vi "GetControllerTemp.vi"(8 "error in (no error)":errorcluster, 11 "SM1000-control in":T1) -> (0 "error out":errorcluster, 2 "Controller temperature":dbl, 3 "SM1000-control out":T1)   [LabVIEW 2013, in "SLMControl.lvlib" / "SM1000.lvclass"]
doc: "Returns the current temperature of the EC1000 board in degrees Celsius.\n\nCommand: \"GetControllerTemp\" or 29\nReturns: floats"
uses:
  SM1000.lvclass
  Object-reference.ctl
  SM1000.lvclass/SM1000.ctl
  Custom-errors.ctl
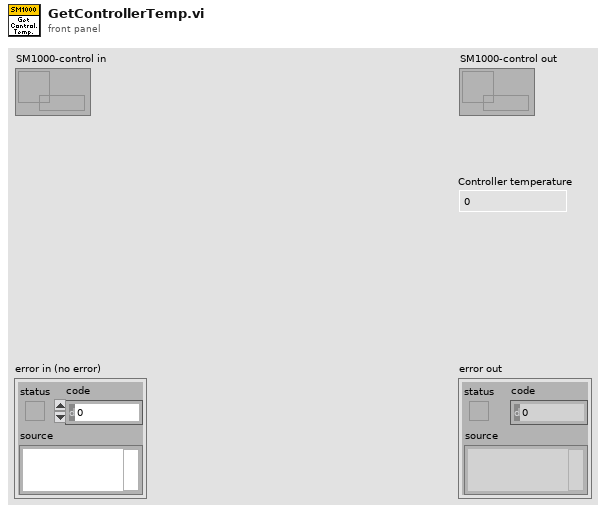
[diagram p1: front panel]
types:
  T1 = typedef "SLMControl.lvlib/SM1000.lvclass/Object-reference.ctl" = refnum<data-value>
  T2 = typedef "SLMControl.lvlib/SM1000.lvclass/Custom-errors.ctl" = enum16{"No error", "Not implemented", "Command not recognized", "Invalid input", "No connection", "Timeout", "Resource not loaded"}
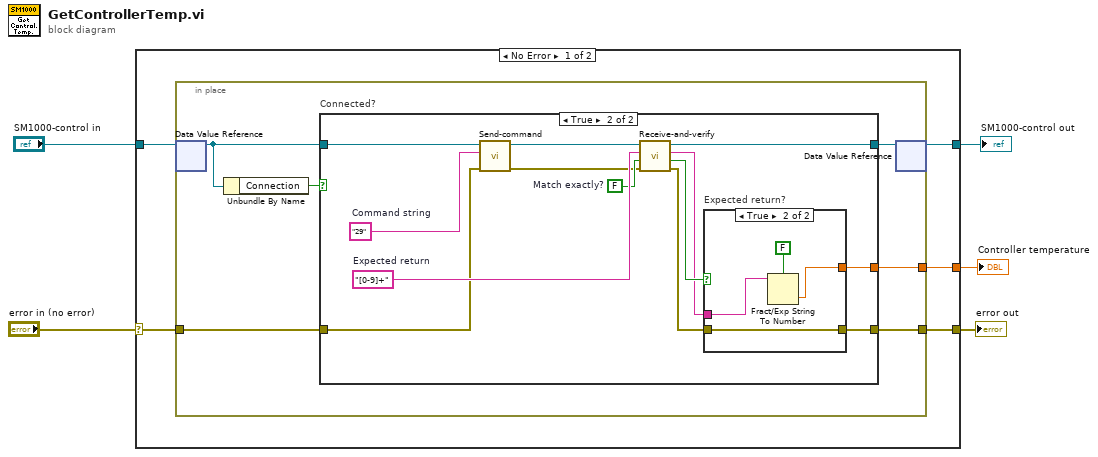
[diagram p0: block diagram]
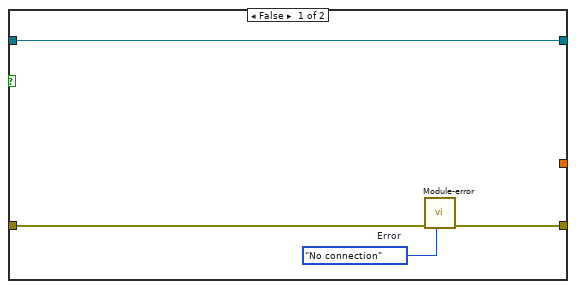
[diagram p2: hidden frame]
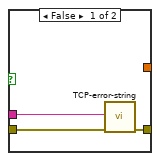
[diagram p3: hidden frame]
diagram:
  n1 = case shown="No Error" "error in (no error)" {
    selector: "error in (no error)" -> [w8 w42]
    tunnel: [w7 w42] -> w4
    tunnel: [w9 w41] -> w2
    tunnel: "SM1000-control in" -> [w10 w41]
    tunnel: [w6 _] -> w1
    frame No Error {
      n2 = in-place {
        in-place-border: w8 -> [w16]
        in-place-border: [w13] -> w7
        in-place-border: [w11] -> w6
        n3 = in-place-dvr #1(w10) -> (w14:refnum<class "SM1000.lvclass">)  [unwired: 1 out]
        n4 = Unbundle By Name(w14) -> ("Connection"=w15:bool)
        n5 = case "Connected?" shown="True" w15 {
          tunnel: w16 -> [w20 w25]
          tunnel: w14 -> [w18 w33]
          tunnel: [w19 w23] -> w13
          tunnel: [w18 w22] -> w12
          tunnel: [_ w21] -> w11
          frame False {
            w17 = Custom-errors."No connection"  # Error
            n6 = call "Module-error.vi"("Error"=w17, "error in (no error)"=w20) -> ("error out"=w19:errorcluster)  [unwired: 9 in]
          }
          frame True {
            w29 = FALSE  # Match exactly?
            w30 = "[0-9]+"  # Expected return
            w31 = "29"  # Command string
            n7 = call "Send-command.vi"("error in (no error)"=w25, "Command string"=w31, "SM1000-control in"=w33) -> ("error out"=w28:errorcluster, "SM1000-control out"=w32:refnum<class "SM1000.lvclass">)  [unwired: 7 in]
            n8 = call "Receive-and-verify.vi"("error in (no error)"=w28, "Match exactly?"=w29, "Expected return string"=w30, "SM1000-control in"=w32) -> ("error out"=w24:errorcluster, "Verified?"=w27:bool, "Return string"=w26:string, "SM1000-control out"=w22:refnum<class "SM1000.lvclass">)  [unwired: 4 in]
            n9 = case "Expected return?" shown="True" w27 {
              tunnel: w26 -> [w36 w39]
              tunnel: w24 -> [w35 w40]
              tunnel: [w34 w40] -> w23
              tunnel: [_ w37] -> w21
              frame False {
                n10 = call "TCP-error-string.vi"("error in (no error)"=w35, "Retun code"=w36) -> ("error out"=w34:errorcluster)  [unwired: 9 in]
              }
              frame True {
                n11 = Fract/Exp String To Number(use system decimal point (T)=FALSE, string=w39) -> (number=w37:dbl)  [unwired: 2 in, 1 out]
              }
            }
          }
        }
        n12 = in-place-dvr #1(w12) -> (w9:T1)  [unwired: 1 out]
      }
    }
    frame Error {
    }
  }
  "error out" <- w4
  "SM1000-control out" <- w2
  "Controller temperature" <- w1
